vi "Read Rx Values Until Equal.vi"(4 "tolerance (0.01)":dbl=0.01, 6 "expected values":dbl[](array[numeric]), 7 "timeout (1000 ms)":i32=1000, 8 "error in":errorcluster, 10 "Rx aliases":string[](array[string]), 11 "workspace manager in":T1) -> (0 "error out":errorcluster, 2 "values equal expected":bool, 3 "workspace manager out":T1)   [LabVIEW 2017, in "VeriStandTestUtilities.lvlib"]
uses:
  VeriStandTestUtilities.lvlib
  <vilib>/NI Veristand/Execution/Workspace/WorkspaceAPI.ctl
  NationalInstruments.VeriStand.ClientAPI
  <vilib>/NI Veristand/Execution/Workspace/NI VeriStand - Get Multiple Channel Values.vi
  <vilib>/NI VeriStand/Execution/Workspace/NI_VS Workspace ExecutionAPI.lvlib
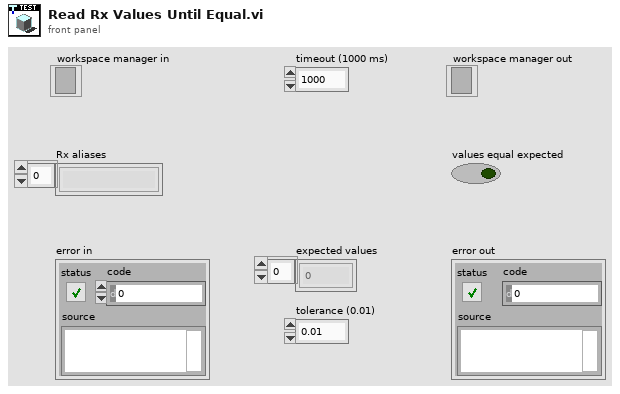
[diagram p1: front panel]
types:
  T1 = typedef "NI_VS Workspace ExecutionAPI.lvlib/WorkspaceAPI.ctl" = refnum<k24>
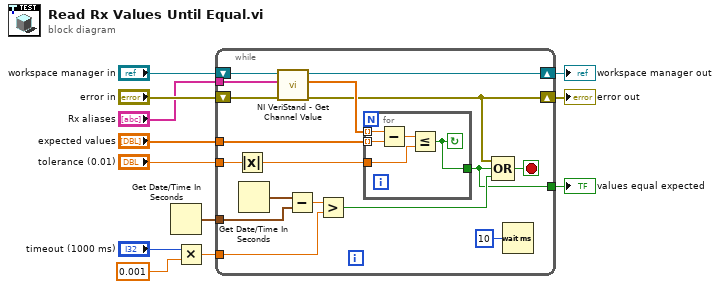
[diagram p0: block diagram]
diagram:
  n1 = Get Date/Time In Seconds() -> (seconds since 1Jan1904=w9:timestamp)
  n2 = Multiply(x="timeout (1000 ms)", y=0.001) -> (x*y=w11:dbl)
  n3 = while {
    tunnel: "Rx aliases" -> [w29]
    shift-right: [w24] -> w3
    shift-left: "error in" -> [w27]
    tunnel: "expected values" -> [w25]
    tunnel: w9 -> [w22]
    tunnel: w11 -> [w20]
    tunnel: [w16] -> w12
    shift-right: [w15] -> w2
    shift-left: "workspace manager in" -> [w28]
    tunnel: "tolerance (0.01)" -> [w14]
    stop <- w18 stop-if-true
    n4 = Absolute Value(x=w14) -> (abs(x)=w13:dbl)
    n5 = Get Date/Time In Seconds() -> (seconds since 1Jan1904=w23:timestamp)
    n6 = call-poly <vilib>:"NI VeriStand - Get Channel Value.vi"("error in (no error)"=w27, "Channels"=w29, "WorkspaceManager in"=w28) -> ("error out"=w24:errorcluster, "Values"=w26:dbl[], "WorkspaceManager out"=w15:T1)  [unwired: 6 in]
    n7 = Subtract(x=w23, y=w22) -> (x-y=w21:dbl)
    n8 = Greater?(x=w21, y=w20) -> (0:w19:bool)
    n9 = for {
      tunnel: w26 -> [w33] mode=indexing
      tunnel: w25 -> [w34] mode=indexing
      tunnel: [w30] -> w16
      tunnel: w13 -> [w31]
      stop <- w30 continue-if-true
      n10 = Subtract(x=w33, y=w34) -> (x-y=w32:dbl)
      n11 = Less Or Equal?(x=w32, y=w31) -> (x <= y?=w30:bool)
    }
    n12 = Compound Arithmetic op=OR(w24, w16, w19) -> (w18:bool)
    n13 = Wait (ms)(milliseconds to wait=u32 10) -> ()  [unwired: 1 out]
  }
  "values equal expected" <- w12
  "error out" <- w3
  "workspace manager out" <- w2
